vi "Set_SN_Coords.vi"(8 "Coords EPOCH":dbl, 9 "input_DEC":dbl format="%<%H:%M:%S>t", 10 "input_RA":dbl format="%<%H:%M:%S%1u>t", 11 "ScopeSim._Telescope":refnum<k7>) -> (0 "precessed_DEC":dbl format="%<%H:%M:%S%1u>t", 3 "precessed_RA":dbl format="%<%H:%M:%S%2u>t")   [LabVIEW 2011]
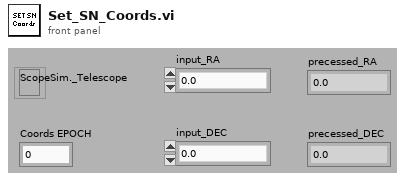
[diagram p1: front panel]
types:
  T1 = typedef "LVDateTimeRec.ctl" = cluster{"fractional second":dbl, "second":i32, "minute":i32, "hour":i32, "day of month":i32, "month":i32, "year":i32, "day of week":i32, "day of year":i32, "DST":i32}
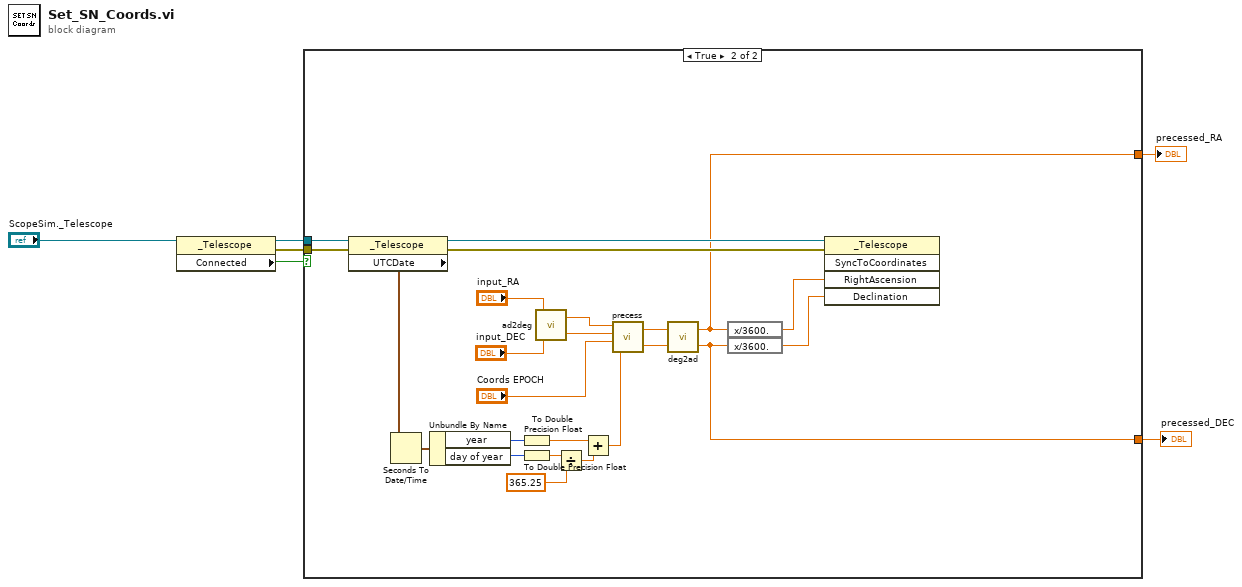
[diagram p0: block diagram]
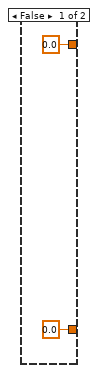
[diagram p2: hidden frame]
diagram:
  n1 = property class="_Telescope"(reference="ScopeSim._Telescope") -> (reference out=w6:refnum<k7>, error out=w4:errorcluster, "Connected"=w5:bool)  [unwired: 1 in]
  n2 = case shown="True" w5 {
    tunnel: w6 -> [_ w32]
    tunnel: w4 -> [_ w22]
    tunnel: [0.0 ("RA (sec)") w9] -> w3
    tunnel: [0.0 ("DEC (sec)") w10] -> w2
    frame False {
    }
    frame True {
      n3 = property class="_Telescope"(reference=w32, error in=w22) -> (reference out=w24:refnum<k7>, error out=w21:errorcluster, "UTCDate"=w23:timestamp)
      n4 = Seconds To Date/Time(time stamp (now)=w23) -> (date time rec=w25:T1)  [unwired: 1 in]
      n5 = Unbundle By Name(w25) -> ("year"=w28:i32, "day of year"=w26:i32)
      n6 = To Double Precision Float(number=w28) -> (double precision float=w30:dbl)
      n7 = To Double Precision Float(number=w26) -> (double precision float=w27:dbl)
      n8 = call "ad2deg.vi"("DEC (sec)"="input_DEC", "RA (sec)"="input_RA") -> ("DEC (°)"=w17:dbl, "RA (°)"=w18:dbl)
      n9 = Divide(x=w27, y=365.25) -> (x/y=w31:dbl)
      n10 = Add(x=w30, y=w31) -> (x+y=w15:dbl)
      n11 = call "precess.vi"("Eq2"=w15, "Eq1"="Coords EPOCH", "DEC 1"=w17, "RA 1"=w18) -> ("DEC 2"=w14:dbl, "RA 2"=w13:dbl)
      n12 = call "deg2ad.vi"("DEC (°)"=w14, "RA (°)"=w13) -> ("DEC (°)"=w10:dbl, "RA (sec)"=w9:dbl)
      n13 = expression code="x/3600."(w9) -> (w11:dbl)
      n14 = expression code="x/3600."(w10) -> (w12:dbl)
      n15 = invoke class="_Telescope" method="SyncToCoordinates"(reference=w24, error in=w21, "RightAscension"=w11, "Declination"=w12) -> ()  [unwired: 1 in, 5 out]
    }
  }
  "precessed_RA" <- w3
  "precessed_DEC" <- w2
